vi "LinearExtensionPixelValues-1.vi"(8 "error in":errorcluster, 11 "[IN] Max Projected Image":T1) -> (0 "error out":errorcluster, 3 "[OUT] Processed Image":T1)   [LabVIEW 2020]
doc: "Draws the cross for showing a center of mass"
uses:
  <vilib>/vision/Image Controls.llb/IMAQ Image.ctl
  <vilib>/vision/NI_Vision_Development_Module.lvlib
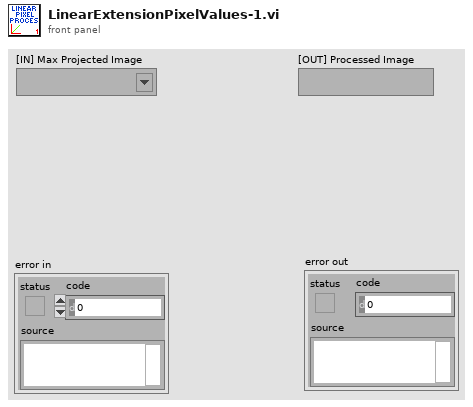
[diagram p1: front panel]
types:
  T1 = typedef "IMAQ Image.ctl" = refnum<image>
  T2 = cluster{"histogram":u32[], "Minimal Value":sgl, "Maximal Value":sgl, "Starting Value":sgl, "Interval Width":sgl, "Mean Value":sgl, "Standard  Variation":sgl, "Area (pixels)":i32}
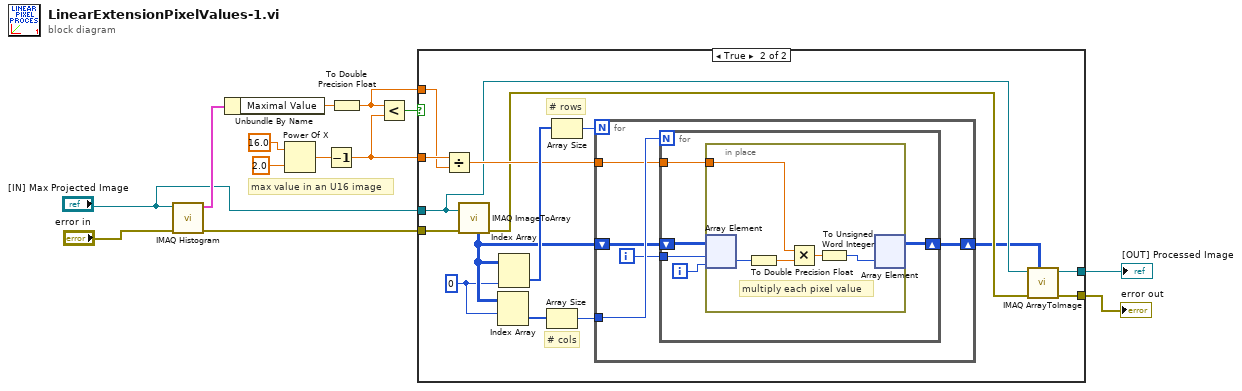
[diagram p0: block diagram]
diagram:
  # "max value in an U16 image"
  n1 = call "IMAQ Histogram"("error in (no error)"="error in", "Image"="[IN] Max Projected Image") -> ("error out"=w2:errorcluster, "Histogram Report"=w3:T2)  [unwired: 8 in]
  n2 = Unbundle By Name(w3) -> ("Maximal Value"=w10:sgl)
  n3 = Power Of X(1:2.0 ("x"), 2:16.0 ("y")) -> (0:w11:dbl)
  n4 = Decrement(x=w11) -> (x-1=w8:dbl)
  n5 = To Double Precision Float(number=w10) -> (double precision float=w7:dbl)
  n6 = Less?(x=w7, y=w8) -> (x < y?=w9:bool)
  n7 = case shown="True" w9 {
    tunnel: w8 -> [_ w30]
    tunnel: w7 -> [_ w29]
    tunnel: "[IN] Max Projected Image" -> [w15 w19]
    tunnel: w2 -> [w14 w28]
    tunnel: [w15 w17] -> w6
    tunnel: [w14 w16] -> w5
    frame False {
    }
    frame True {
      w22 = 0
      # "# cols"
      # "# rows"
      n8 = Divide(x=w30, y=w29) -> (x/y=w21:dbl)
      n9 = call "IMAQ ImageToArray"("error in (no error)"=w28, "Image"=w19) -> ("Image Pixels (U16)"=w25:u16[][], "error out"=w20:errorcluster)  [unwired: 2 in, 3 out]
      n10 = Index Array(array=w25, index (row)=w22) -> (element=w24:u16[])  [unwired: 1 in]
      n11 = Index Array(array=w25, index (col)=w22) -> (element=w27:u16[])  [unwired: 1 in]
      n12 = Array Size(array=w24) -> (size(s)=w23:i32)
      n13 = Array Size(array=w27) -> (size(s)=w26:i32)
      n14 = for {
        N: w26 -> [_]
        shift-right: [w31] -> w18
        shift-left: w25 -> [w34]
        tunnel: w23 -> [w35]
        tunnel: w21 -> [w33]
        i -> [w32]
        n15 = for {
          N: w35 -> [_]
          shift-right: [w36] -> w31
          shift-left: w34 -> [w40]
          tunnel: w33 -> [w37]
          tunnel: w32 -> [w39]
          i -> [w38]
          n16 = in-place {
            in-place-border: w37 -> [w43]
            # "multiply each pixel value"
            n17 = in-place-array #1(w40, w39, w38) -> (w45:u16)
            n18 = To Double Precision Float(number=w45) -> (double precision float=w44:dbl)
            n19 = Multiply(x=w43, y=w44) -> (x*y=w42:dbl)
            n20 = To Unsigned Word Integer(number=w42) -> (unsigned 16bit integer=w41:u16)
            n21 = in-place-array #1(w41) -> (w36:u16[][])  [unwired: 2 out]
          }
        }
      }
      n22 = call "IMAQ ArrayToImage"("Image Pixels (U16)"=w18, "error in (no error)"=w20, "Image"=w19) -> ("error out"=w16:errorcluster, "Image Out"=w17:T1)  [unwired: 7 in]
    }
  }
  "error out" <- w5
  "[OUT] Processed Image" <- w6
